vi "process.vi"(8 "error in (no error)":errorcluster, 11 "Session in":refnum<class "Session.lvclass">) -> (0 "error out":errorcluster, 3 "Session out":refnum<class "Session.lvclass">)   [LabVIEW 2013, in "MQTT Server.lvlib" / "Session.lvclass"]
uses:
  Session.lvclass
  Control Packets/ControlPacket/ControlPacket.lvclass
  Session.lvclass/Session.ctl
  Connection/TCPConnection.lvclass
panel:
  out "Last Request":timestamp
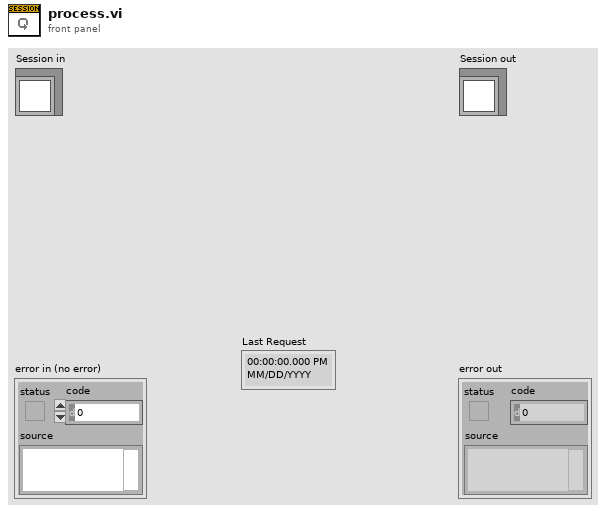
[diagram p1: front panel]
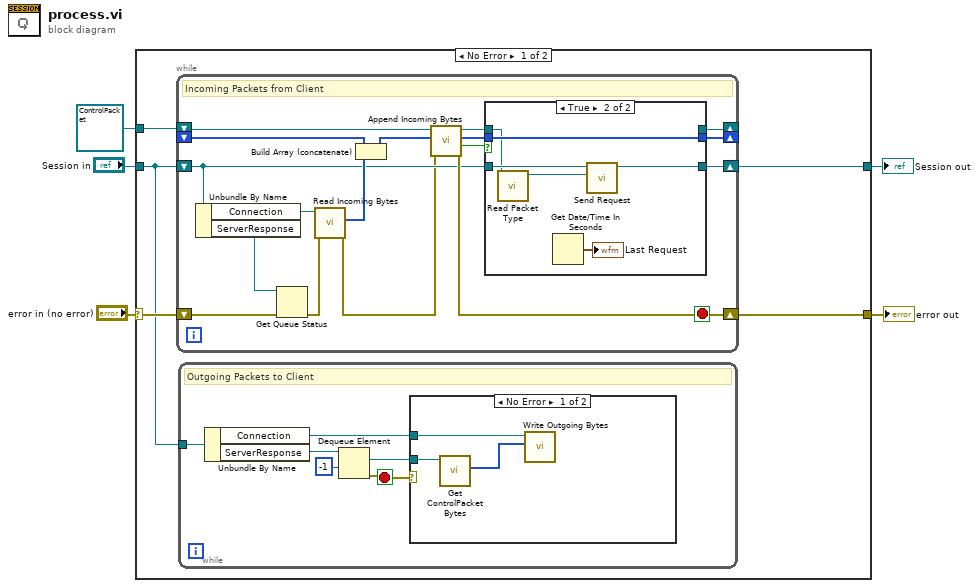
[diagram p0: block diagram]
diagram:
  n1 = case shown="No Error" "error in (no error)" {
    selector: "error in (no error)" -> [w9 w47]
    tunnel: [w8 w47] -> w2
    tunnel: [w10 w46] -> w4
    tunnel: "Session in" -> [w6 w46]
    tunnel: refnum<class "ControlPacket.lvclass"> refnum ("Incomplete ControlPacket") -> [w7 _]
    frame No Error {
      n2 = while {
        shift-right: [w25] -> w10
        shift-left: w6 -> [w24]
        shift-right: [w26] -> w8
        shift-left: w9 -> [w21]
        shift-right: [w32] -> _
        shift-left: w7 -> [w36]
        shift-right: [w30] -> _
        shift-left: _ -> [w29]
        stop <- w26 stop-if-true
        # "Incoming Packets from Client"
        n3 = Unbundle By Name(w24) -> ("Connection"=w35:refnum<class "TCPConnection.lvclass">, "ServerResponse"=w22:refnum<queue>)
        n4 = Get Queue Status(queue=w22, error in (no error)=w21) -> (error out=w20:errorcluster)  [unwired: 1 in, 7 out]
        n5 = call "Read Incoming Bytes.vi"("error in (no error)"=w20, "TCPConnection in"=w35) -> ("error out"=w23:errorcluster, "Bytes"=w28:u8[])  [unwired: 7 in, 1 out]
        n6 = Build Array (concatenate)(w29, w28) -> (w27:u8[])
        n7 = call "Append Incoming Bytes.vi"("error in (no error)"=w23, "Incoming Packets"=w27, "Incomplete ControlPacket"=w36) -> ("error out"=w26:errorcluster, "Complete Packet"=w34:bool, "Remaining Packets"=w31:u8[], "ControlPacket"=w33:refnum<class "ControlPacket.lvclass">)  [unwired: 5 in]
        n8 = case shown="True" w34 {
          tunnel: w33 -> [w39 w41]
          tunnel: [w39 _] -> w32
          tunnel: w31 -> [w38 w44]
          tunnel: [w38 w44] -> w30
          tunnel: [w37 w42] -> w25
          tunnel: w24 -> [w37 w43]
          frame False {
          }
          frame True {
            n9 = call "Read Packet Type.vi"("ControlPacket in"=w41) -> ("ControlPacket out"=w40:refnum<class "ControlPacket.lvclass">)  [unwired: 9 in, 1 out]
            n10 = Get Date/Time In Seconds() -> (seconds since 1Jan1904=→"Last Request":timestamp)
            n11 = call "Send Request.vi"("ServerRequest"=w40, "Session in"=w43) -> ("Session out"=w42:refnum<class "Session.lvclass">)  [unwired: 8 in, 1 out]
          }
        }
      }
      n12 = while {
        tunnel: w6 -> [w16]
        stop <- w12 stop-if-true
        # "Outgoing Packets to Client"
        n13 = Unbundle By Name(w16) -> ("Connection"=w11:refnum<class "TCPConnection.lvclass">, "ServerResponse"=w15:refnum<queue>)
        n14 = Dequeue Element(queue=w15, timeout in ms (-1)=-1) -> (element=w13:refnum<class "ControlPacket.lvclass">, error out=w12:errorcluster)  [unwired: 1 in, 2 out]
        n15 = case shown="No Error" w12 {
          tunnel: w13 -> [w19 _]
          tunnel: w11 -> [w18 _]
          frame No Error {
            n16 = call "Get ControlPacket Bytes.vi"("ControlPacket"=w19) -> ("Bytes Stream"=w17:u8[])  [unwired: 8 in, 2 out]
            n17 = call "Write Outgoing Bytes.vi"("Bytes"=w17, "TCPConnection in"=w18) -> ()  [unwired: 8 in, 2 out]
          }
          frame Error {
          }
        }
      }
    }
    frame Error {
    }
  }
  "error out" <- w2
  "Session out" <- w4
